vi "CMFB diagnostic.vi"() -> ()   [LabVIEW 2019]
uses:
  <vilib>/Platform/TimedLoop/XDataNode/timing_clust.ctl
  <vilib>/Platform/TimedLoop/XDataNode/nitl_modes.ctl
  <vilib>/Platform/TimedLoop/XDataNode/wakeup.ctl
  <vilib>/rvi/FXPMathLib/FxpDiv/subVIs/nifxpmath_Div_SimConfig.ctl
  <vilib>/rvi/Emulation/niFpgaGetClockAttributes.vi
  <vilib>/rvi/Emulation/niFpgaSctlEmulationGetInTimedLoop.vi
  <vilib>/rvi/Emulation/niFpgaEmulationReportErrorSimple.vi
  <vilib>/rvi/Emulation/niFpgaProcessEmulError.vi
  <vilib>/rvi/Emulation/niFpgaCriticalErrorInLSC.vi
  <vilib>/rvi/FXPMathLib/FxpDiv/simVIs/DllFxpDivTemp_sub.vi
  <vilib>/Platform/TimedLoop/XDataNode/XDataNode.xnode
  <vilib>/rvi/FXPMathLib/FxpDiv/XNode/nifxpmath_Div.xnode
  <vilib>/Platform/TimedLoop/XDataNode/XDNodeRunTimeDep.lvlib
panel:
  in  "Wait Low (ms)":u32=100
  in  "Wait High (ms)":u32=100
  out "Freq":bool=TRUE
  out "flow freq":fxp<+/-,28,17>=5.0
  in  "Max Period (ticks)":u32=40000000
  out "diag freq":fxp<+/-,32,32>=4000008.0
  out "Diagnostic (duty)":fxp<+/-,28,17>=65535.99951171875
  in  "Diagnostic Filter":u16=500
  in  "Invert Diagnostic":bool
  in  "Diagnostic Freq Coeff":i32=40000
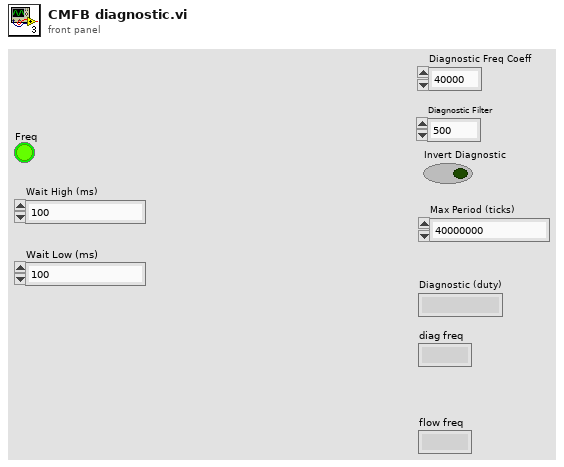
[diagram p1: front panel]
types:
  T1 = typedef "XDNodeRunTimeDep.lvlib/timing_clust.ctl" = cluster{"Expected End [f-1]":u64, "Actual End [f-1]":u64, "Finished Late? [f-1]":bool, "Expected End [i-1]":u64, "Actual End [i-1]":u64, "Finished Late? [i-1]":bool, "Expected Start [i]":u64, "Actual Start [i]":u64, "Expected Start [f]":u64, "Actual Start [f]":u64, "Source Name":string, "Structure Name":string, "Period":i64, "Deadline":i64, "Offset":i64, "Start":i64, "Priority":i32, "Timeout":i32, "Mode":T2, "Wakeup Reason":T3, "Error":errorcluster, "Source Type":string, "Secondary Source Type":string, "Global End Time":u64, "Global Start Time":u64, "Frame Duration":u64, "Iteration Duration":u64, "Assigned CPU":i32, "I/O Scan Engine Mode":u32}
  T2 = typedef "XDNodeRunTimeDep.lvlib/nitl_modes.ctl" = enum32{"No Change", "Process missed periods, maintain original phase", "Discard missed periods, maintain original phase", "Process missed periods, ignore original phase", "Discard missed periods, ignore original phase"}
  T3 = typedef "XDNodeRunTimeDep.lvlib/wakeup.ctl" = enum32{"Normal", "Aborted", "Asynchronous wakeup", "Timing source error", "Timed loop error", "Timeout"}
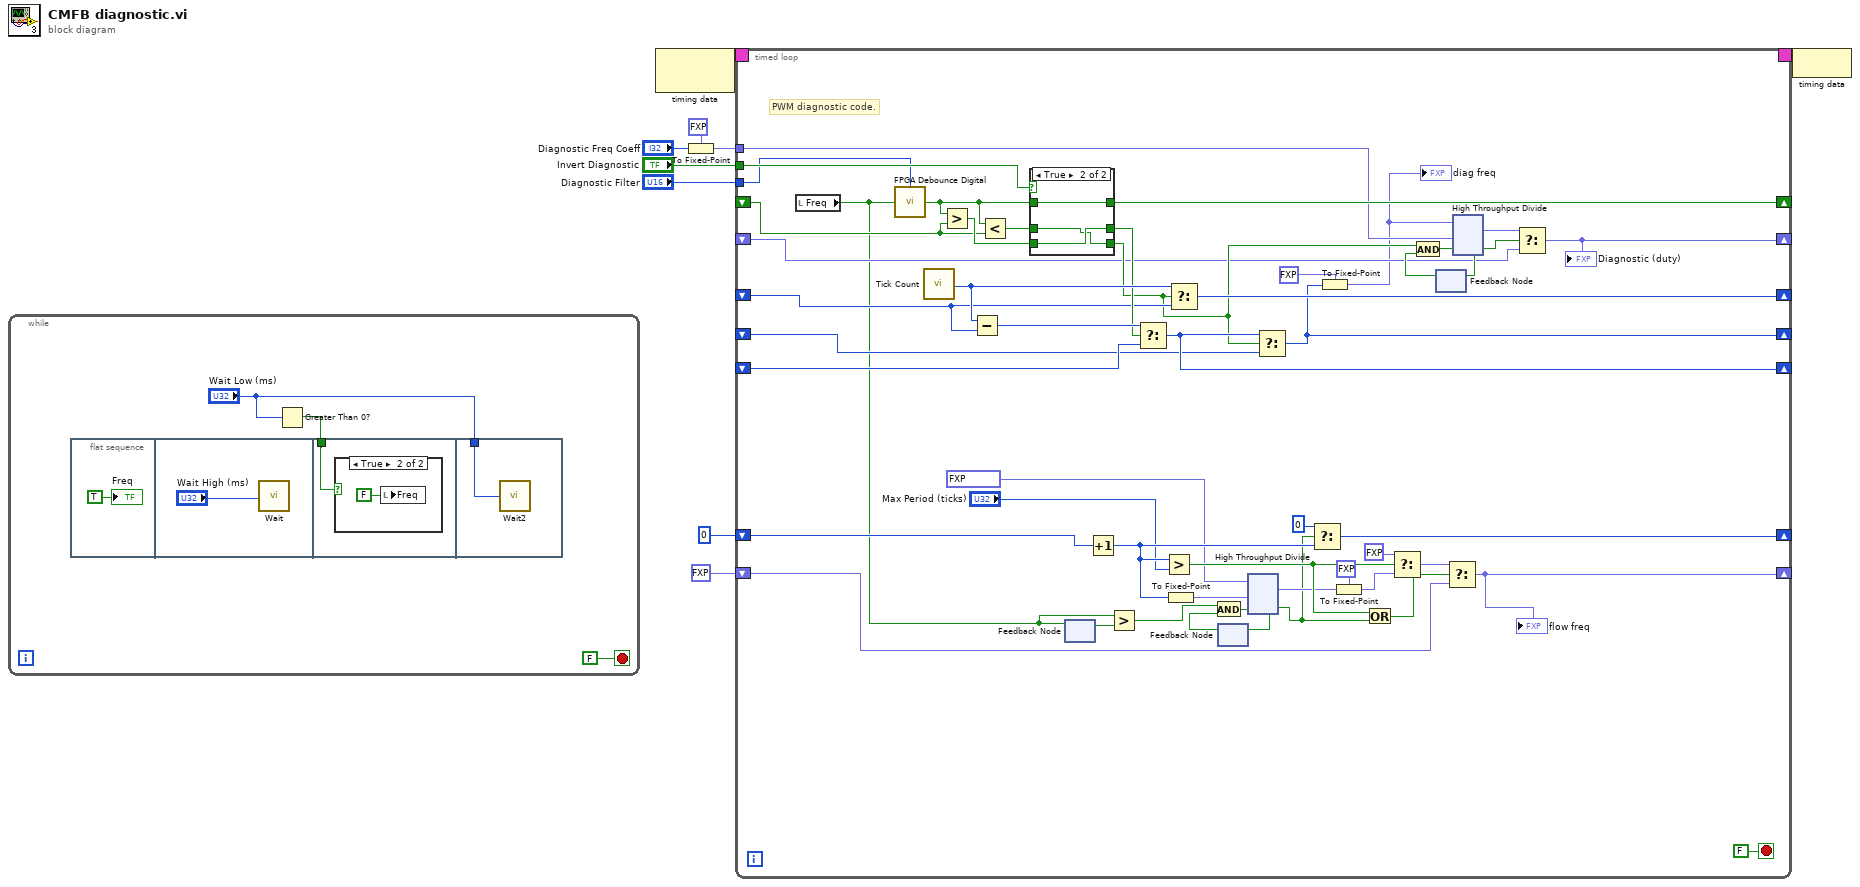
[diagram p0: block diagram]
diagram:
  n1 = while {
    stop <- FALSE stop-if-true
    n2 = flat-sequence {
      tunnel: w10 -> [w15]
      tunnel: "Wait Low (ms)" -> [w17]
      frame #0 {
        "Freq" <- TRUE
      }
      frame #1 {
        n3 = call "Wait"("Count(mSec)"="Wait High (ms)") -> ()  [unwired: 1 out]
      }
      frame #2 {
        n4 = case shown="True" w15 {
          frame False {
          }
          frame True {
            n5 = local write "Freq"(FALSE ("Freq")) -> ()
          }
        }
      }
      frame #3 {
        n6 = call "Wait2"("Count(mSec)"=w17) -> ()  [unwired: 1 out]
      }
    }
    n7 = Greater Than 0?(x="Wait Low (ms)") -> (x > 0?=w10:bool)
  }
  n8 = node-c288() -> (w9:T1)  [unwired: 1 in]
  n9 = To Fixed-Point(fixed-point type=fxp<+/-,32,32> 0.0 ("s? t:f"), number="Diagnostic Freq Coeff") -> (fixed-point=w5:fxp<+/-,32,32>)
  n10 = timed-loop {
    shift-right: [w62] -> _
    shift-left: _ -> [w61]
    shift-right: [w60] -> _
    shift-left: _ -> [w59]
    shift-right: [w53] -> _
    shift-left: _ -> [w58]
    shift-right: [w51] -> _
    shift-left: _ -> [w52]
    tunnel: w5 -> [w44]
    timing: w9 -> [_]
    timing-out: [_] -> w8
    tunnel: "Invert Diagnostic" -> [w45]
    shift-right: [w46] -> _
    shift-left: _ -> [w47]
    tunnel: "Diagnostic Filter" -> [w42]
    shift-right: [w22] -> _
    shift-left: u32 0 ("f") -> [w19]
    shift-right: [w21] -> _
    shift-left: fxp<+/-,28,17> 0.0 ("AI0") -> [w20]
    stop <- FALSE stop-if-true
    # "PWM diagnostic code."
    n11 = local read "Freq"() -> (w18:bool)
    n12 = call "FPGA Debounce Digital.vi"("Input Signal"=w18, "Cycles to Filter"=w42) -> ("Output Filtered Signal"=w43:bool)
    n13 = call "Tick Count"() -> ("Tick Count(Ticks)"=w68:u32)
    n14 = Greater?(x=w43, y=w59) -> (0:w65:bool)
    n15 = Subtract(x=w68, y=w61) -> (x-y=w67:u32)
    n16 = Less?(x=w43, y=w59) -> (x < y?=w66:bool)
    n17 = case shown="True" w45 {
      tunnel: w66 -> [w129 w131]
      tunnel: w65 -> [w128 w132]
      tunnel: [w129 w132] -> w64
      tunnel: [w128 w131] -> w50
      tunnel: w43 -> [w127 w130]
      tunnel: [w127 w130] -> w60
      frame False {
      }
      frame True {
      }
    }
    n18 = feedback #1() -> (w40:bool)  [unwired: 1 in]
    n19 = feedback-in #1(w18) -> ()
    n20 = Increment(x=w19) -> (x+1=w37:u32)
    n21 = Greater?(x=w18, y=w40) -> (0:w25:bool)
    n22 = Select(t=w67, s=w64, f=w58) -> (s? t:f=w53:u32)
    n23 = Greater?(x=w37, y="Max Period (ticks)") -> (0:w39:bool)
    n24 = To Fixed-Point(number=w37) -> (fixed-point=w36:fxp<+,32,32>)  [unwired: 1 in]
    n25 = Select(t=w68, s=w50, f=w61) -> (s? t:f=w62:u32)
    n26 = feedback #2() -> (w26:bool)  [unwired: 1 in]
    n27 = And(x=w25, y=w26) -> (x .and. y?=w27:bool)
    n28 = xnode "High Throughput Divide"("x"=fxp<+,32,32> 40000000.0, "y"=w36, "input valid"=w27) -> ("x/y"=w33:fxp<+,28,17>, "output valid"=w29:bool, "ready for input"=w28:bool)  [unwired: 1 in]
    n29 = feedback-in #2(w28) -> ()
    n30 = Select(t=w53, s=w50, f=w52) -> (s? t:f=w51:u32)
    n31 = Select(t=u32 0 ("f"), s=w29, f=w37) -> (s? t:f=w22:u32)
    n32 = To Fixed-Point(fixed-point type=fxp<+/-,32,32> 0.0 ("s? t:f"), number=w51) -> (fixed-point=w41:fxp<+/-,32,32>)
    "diag freq" <- w41
    n33 = To Fixed-Point(fixed-point type=fxp<+/-,28,17> 0.0 ("AI0"), number=w33) -> (fixed-point=w31:fxp<+/-,28,17>)
    n34 = Or(x=w39, y=w29) -> (x .or. y?=w34:bool)
    n35 = Select(t=fxp<+/-,28,17> 0.0 ("AI0"), s=w39, f=w31) -> (s? t:f=w35:fxp<+/-,28,17>)
    n36 = feedback #3() -> (w54:bool)  [unwired: 1 in]
    n37 = And(x=w50, y=w54) -> (x .and. y?=w55:bool)
    n38 = Select(t=w35, s=w34, f=w20) -> (s? t:f=w21:fxp<+/-,28,17>)
    "flow freq" <- w21
    n39 = xnode "High Throughput Divide"("x"=w41, "y"=w44, "input valid"=w55) -> ("x/y"=w49:fxp<+/-,28,17>, "output valid"=w48:bool, "ready for input"=w56:bool)  [unwired: 1 in]
    n40 = feedback-in #3(w56) -> ()
    n41 = Select(t=w49, s=w48, f=w47) -> (s? t:f=w46:fxp<+/-,28,17>)
    "Diagnostic (duty)" <- w46
  }
  n42 = node-c288(w8) -> ()
